vi "Add Copyright.vi"(8 "error in (no error)":errorcluster, 9 "Delimiter":string, 10 "Copyright":string, 11 "VI in":refnum<class "VI.lvclass">) -> (0 "error out":errorcluster, 3 "VI out":refnum<class "VI.lvclass">)   [LabVIEW 2020, in "VI Properties Editor.lvlib" / "VI.lvclass"]
doc: "Adds <B>Copyright</B> to <B>VI in</B>."
uses:
  VI.lvclass
  Item/Item.lvclass
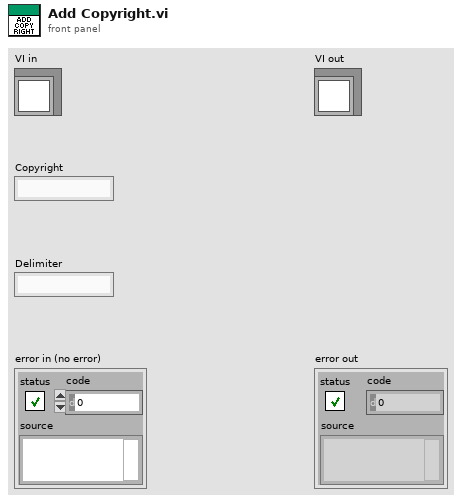
[diagram p1: front panel]
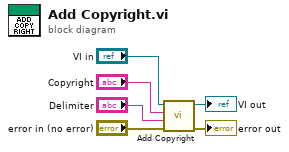
[diagram p0: block diagram]
diagram:
  n1 = call-parent "Add Copyright.vi"("error in (no error)"="error in (no error)", "Delimiter"="Delimiter", "Copyright"="Copyright", "Item in"="VI in") -> ("error out"=→"error out":errorcluster, "Item out"=→"VI out":refnum<class "VI.lvclass">)  [unwired: 6 in]
